vi "oa_Convert Bandwidth to Integration Revolutions.vi"(1 "bandwidth [order]":dbl) -> (0 "integration revolutions":dbl)   [LabVIEW 2017]
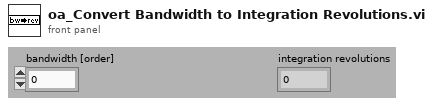
[diagram p1: front panel]
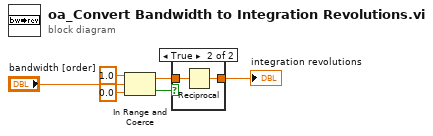
[diagram p0: block diagram]
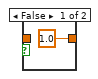
[diagram p2: hidden frame]
diagram:
  n1 = In Range and Coerce(upper limit=1.0, x="bandwidth [order]", lower limit=0.0) -> (coerced(x)=w6:dbl, In Range?=w5:bool)
  n2 = case shown="True" w5 {
    tunnel: w6 -> [_ w9]
    tunnel: [1.0 w8] -> w1
    frame False {
    }
    frame True {
      n3 = Reciprocal(x=w9) -> (1/x=w8:dbl)
    }
  }
  "integration revolutions" <- w1
